vi "ExecuteSequence.vi"(8 "error in (no error)":errorcluster, 11 "Sequence in":refnum<class "Sequence.lvclass">) -> (0 "error out":errorcluster, 1 "Command":string, 2 "SweepProperties":T1, 3 "Sequence out":refnum<class "Sequence.lvclass">, 4 "Sequence is done":bool, 6 "Next Position":T4)   [LabVIEW 2018, in "Sequence.lvclass"]
uses:
  Sequence.lvclass
  SequenceSubvis/PatchNewTestStep.ctl
  SequenceSubvis/RF Direction.ctl
  SequenceSubvis/PolarizationSelect.ctl
  APARMainSubvis/VXM Public API/singleAxisMoveDef.ctl
  APARMainSubvis/VXM Public API/mmWaveAxis.ctl
  Datalog/DatalogSubvis/SearchableTag.ctl
  Support/MessageAPI/UIMessage.ctl
  Sequence.lvclass/Sequence.ctl
  SendMessage/SendMessage.lvclass
  Datalog/DataLog.lvclass
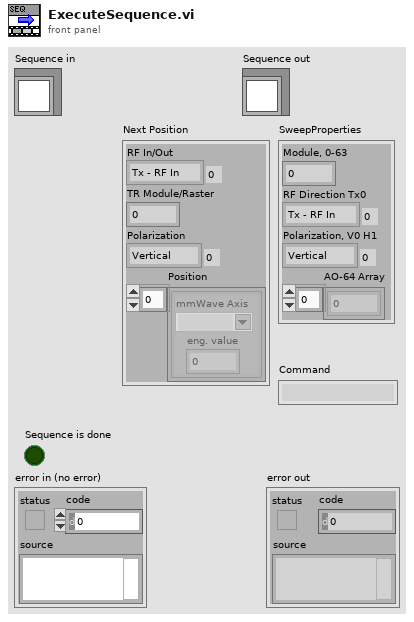
[diagram p1: front panel]
types:
  T1 = typedef "DataLog.lvclass/SearchableTag.ctl" = cluster{"Module, 0-63":i32, "RF Direction Tx0":T2, "Polarization, V0 H1":T3, "AO-64 Array":dbl[]}
  T2 = typedef "RF Direction.ctl" = enum16{"Tx - RF In", "Rx - RF Out"}
  T3 = typedef "PolarizationSelect.ctl" = enum16{"Vertical", "Horizontal"}
  T4 = typedef "PatchNewTestStep.ctl" = cluster{"RF In/Out":T2, "TR Module/Raster":i32, "Polarization":T3, "Position":T5[]}
  T5 = typedef "singleAxisMoveDef.ctl" = cluster{"mmWave Axis":T6, "eng. value":dbl}
  T6 = typedef "mmWaveAxis.ctl" = string
  T7 = typedef "UIMessage.ctl" = cluster{"EventCode":i32, "Numeric":dbl, "String":string, "Variant":variant}
  T8 = typedef "mWaveTestStep.ctl" = cluster{"StepType":T9, "RF In/Out":T2, "Module/Raster":i32, "Polarization":T3, "AO-64 Array":dbl[], "Position":T5[]}
  T9 = typedef "TestStepTypes.ctl" = enum16{"MotionFF-M2", "Motion", "SweepTest", "RasterTest", "Finish", "64ModuleCfg"}
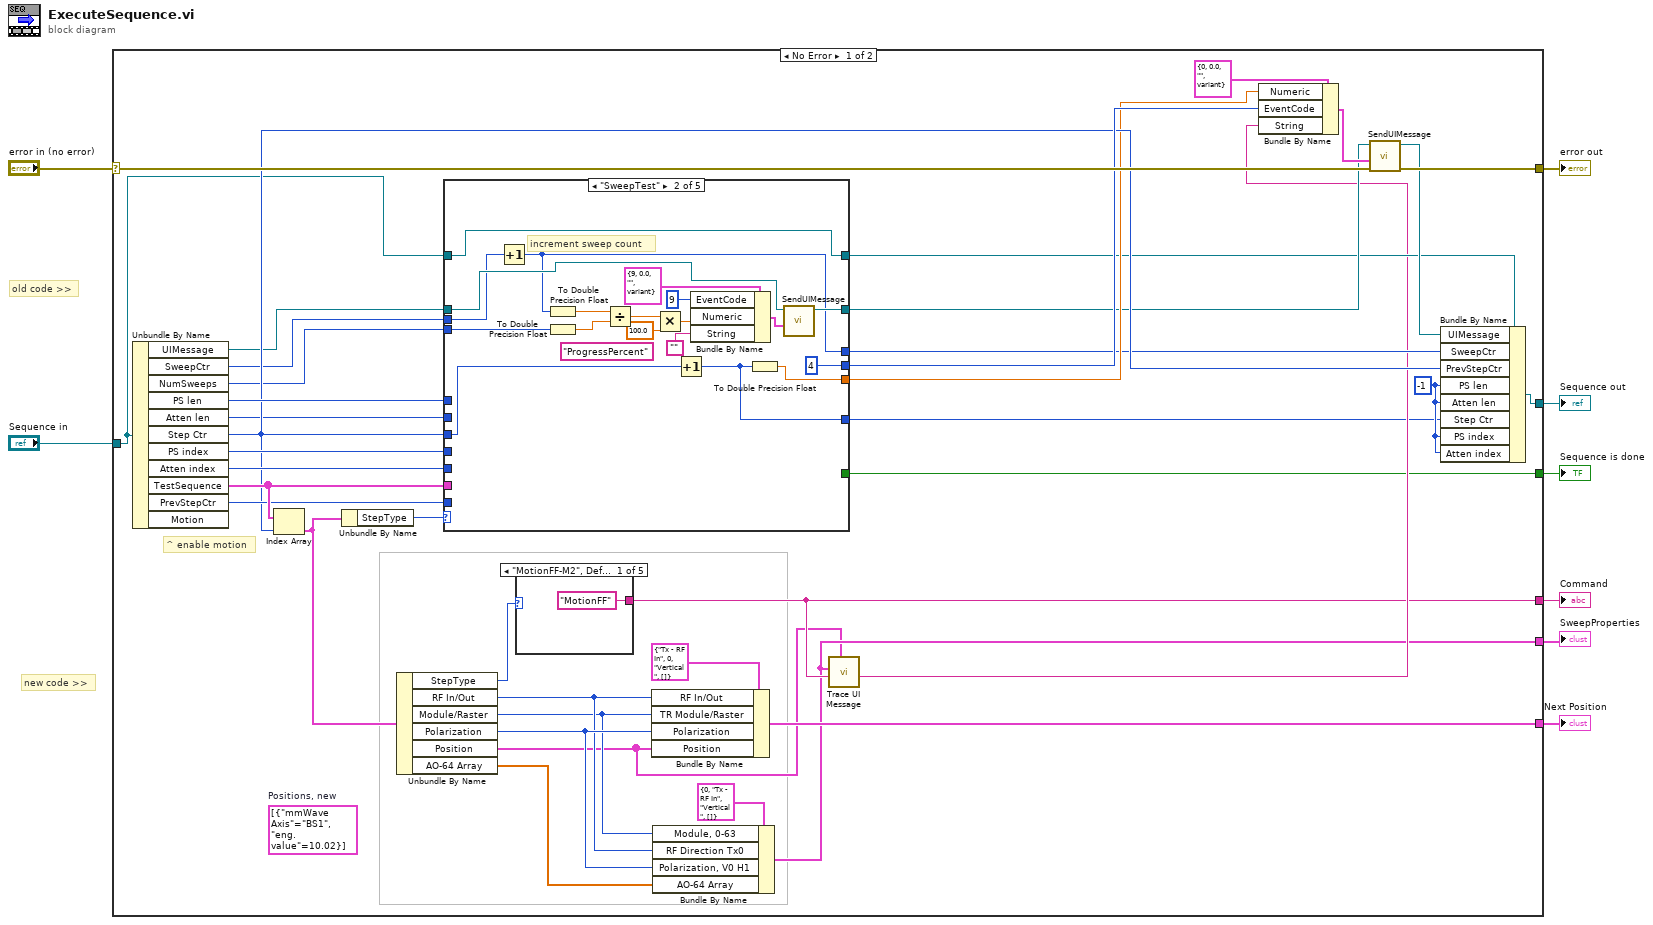
[diagram p0: block diagram]
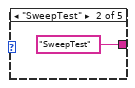
[diagram p2: hidden frame]
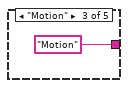
[diagram p3: hidden frame]
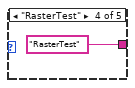
[diagram p4: hidden frame]
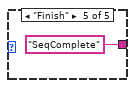
[diagram p5: hidden frame]
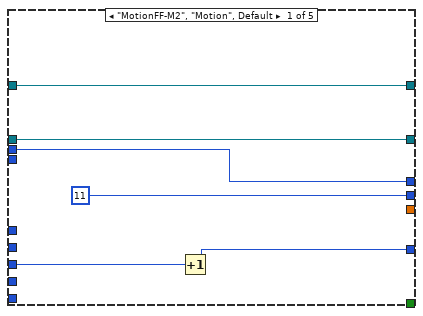
[diagram p6: hidden frame]
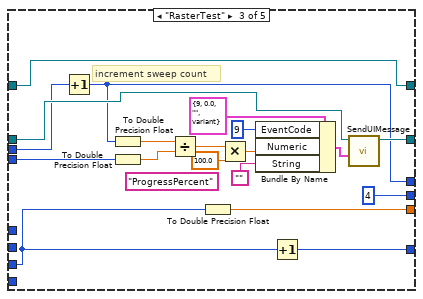
[diagram p7: hidden frame]
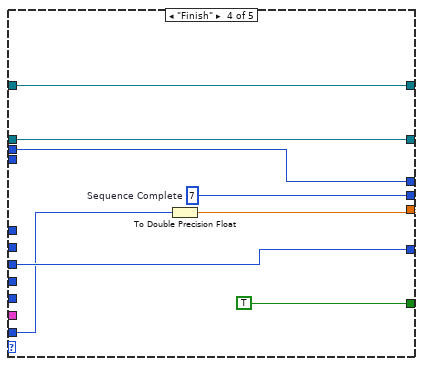
[diagram p8: hidden frame]
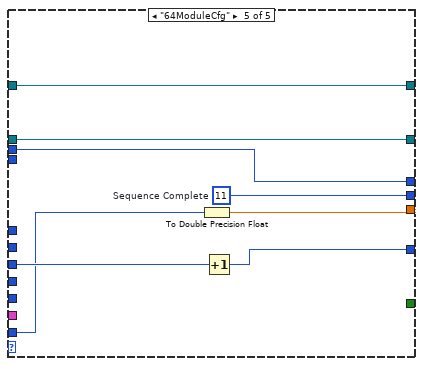
[diagram p9: hidden frame]
diagram:
  # "new code >>"
  # "old code >>"
  n1 = case shown="No Error" "error in (no error)" {
    selector: "error in (no error)" -> [w39 w114]
    tunnel: [w40 w114] -> w7
    tunnel: [w47 w113] -> w5
    tunnel: "Sequence in" -> [w26 w113]
    tunnel: [w12 _] -> w4
    tunnel: [w22 _] -> w3
    tunnel: [w13 _] -> w2
    tunnel: [w11 _] -> w1
    frame No Error {
      (unwired) T5[] [{"mmWave Axis"="BS1", "eng. value"=10.02}]  # Positions, new
      w23 = -1 ("Execution.PS len")
      # "^ enable motion"
      n2 = Unbundle By Name(w26) -> ("UIMessage"=w29:refnum<class "SendMessage.lvclass">, "SweepCtr"=w32:i32, "NumSweeps"=w31:i32, "PS len"=w46:i32, "Atten len"=w34:i32, "Step Ctr"=w35:i32, "PS index"=w45:i32, "Atten index"=w43:i32, "TestSequence"=w44:T8[], "PrevStepCtr"=w36:i32)  [unwired: 1 out]
      n3 = Index Array(array=w44, index=w35) -> (element=w14:T8)
      n4 = Unbundle By Name(w14) -> ("StepType"=w42:T9)
      n5 = Unbundle By Name(w14) -> ("StepType"=w20:T9, "RF In/Out"=w18:T2, "Module/Raster"=w17:i32, "Polarization"=w19:T3, "Position"=w9:T5[], "AO-64 Array"=w10:dbl[])
      n6 = case shown="\"SweepTest\"" w42 {
        tunnel: w45 -> [_ _ _ _ _]
        tunnel: w43 -> [_ _ _ _ _]
        tunnel: w46 -> [_ _ _ _ _]
        tunnel: w35 -> [w54 w76 w94 w102 w110]
        tunnel: [w53 w59 w96 w102 w105] -> w21
        tunnel: w44 -> [_ _ _ _ _]
        tunnel: [11 ("EventCode") 4 ("EventCode") 4 ("EventCode") w104 w112] -> w37
        tunnel: w36 -> [_ _ _ w101 w109]
        tunnel: w34 -> [_ _ _ _ _]
        tunnel: [_ w75 w93 w103 w111] -> w33
        tunnel: w32 -> [w57 w64 w82 w100 w108]
        tunnel: w31 -> [_ w70 w88 _ _]
        tunnel: [w57 w63 w81 w100 w108] -> w30
        tunnel: w29 -> [w56 w65 w83 w99 w107]
        tunnel: [w56 w69 w87 w99 w107] -> w28
        tunnel: w26 -> [w55 w60 w78 w98 w106]
        tunnel: [w55 w60 w78 w98 w106] -> w25
        tunnel: [_ _ _ TRUE _] -> w22
        frame "MotionFF-M2", "Motion", Default {
          n7 = Increment(x=w54) -> (x+1=w53:i32)
        }
        frame "SweepTest" {
          (unwired) "ProgressPercent" ("String")
          # "increment sweep count"
          n8 = Increment(x=w64) -> (x+1=w63:i32)
          n9 = To Double Precision Float(number=w63) -> (double precision float=w73:dbl)
          n10 = To Double Precision Float(number=w70) -> (double precision float=w72:dbl)
          n11 = Divide(x=w73, y=w72) -> (x/y=w68:dbl)
          n12 = Multiply(x=w68, y=100.0) -> (x*y=w66:dbl)
          n13 = Increment(x=w76) -> (x+1=w59:i32)
          n14 = Bundle By Name(cluster=T7 {"EventCode"=9, "Numeric"=0.0, "String"="", "Variant"=variant} ("UIMsg"), "EventCode"=9, "Numeric"=w66, "String"="") -> (w71:T7)
          n15 = To Double Precision Float(number=w59) -> (double precision float=w75:dbl)
          n16 = call-dynamic "SendUIMessage.vi"("UIMsg"=w71, "SendMessage in"=w65) -> ("SendMessage out"=w69:refnum<class "SendMessage.lvclass">)  [unwired: 8 in, 1 out]
        }
        frame "RasterTest" {
          (unwired) "ProgressPercent" ("String")
          # "increment sweep count"
          n17 = Increment(x=w82) -> (x+1=w81:i32)
          n18 = To Double Precision Float(number=w81) -> (double precision float=w91:dbl)
          n19 = To Double Precision Float(number=w88) -> (double precision float=w90:dbl)
          n20 = Divide(x=w91, y=w90) -> (x/y=w86:dbl)
          n21 = To Double Precision Float(number=w94) -> (double precision float=w93:dbl)
          n22 = Multiply(x=w86, y=100.0) -> (x*y=w84:dbl)
          n23 = Bundle By Name(cluster=T7 {"EventCode"=9, "Numeric"=0.0, "String"="", "Variant"=variant} ("UIMsg"), "EventCode"=9, "Numeric"=w84, "String"="") -> (w89:T7)
          n24 = Increment(x=w94) -> (x+1=w96:i32)
          n25 = call-dynamic "SendUIMessage.vi"("UIMsg"=w89, "SendMessage in"=w83) -> ("SendMessage out"=w87:refnum<class "SendMessage.lvclass">)  [unwired: 8 in, 1 out]
        }
        frame "Finish" {
          w104 = 7  # Sequence Complete
          n26 = To Double Precision Float(number=w101) -> (double precision float=w103:dbl)
        }
        frame "64ModuleCfg" {
          w112 = 11  # Sequence Complete
          n27 = To Double Precision Float(number=w109) -> (double precision float=w111:dbl)
          n28 = Increment(x=w110) -> (x+1=w105:i32)
        }
      }
      n29 = case shown="\"MotionFF-M2\", Default" w20 {
        tunnel: ["MotionFF" ("Command") "SweepTest" ("Command") "Motion" ("Command") "RasterTest" ("Command") "SeqComplete" ("Command")] -> w13
        frame "MotionFF-M2", Default {
        }
        frame "SweepTest" {
        }
        frame "Motion" {
        }
        frame "RasterTest" {
        }
        frame "Finish" {
        }
      }
      n30 = Bundle By Name(cluster=T4 {"RF In/Out"=enum."Tx - RF In", "TR Module/Raster"=0, "Polarization"=enum."Vertical", "Position"=[]} ("NewSetup"), "RF In/Out"=w18, "TR Module/Raster"=w17, "Polarization"=w19, "Position"=w9) -> (w12:T4)
      n31 = Bundle By Name(cluster=T1 {"Module, 0-63"=0, "RF Direction Tx0"=enum."Tx - RF In", "Polarization, V0 H1"=enum."Vertical", "AO-64 Array"=[]} ("SweepProperties"), "Module, 0-63"=w17, "RF Direction Tx0"=w18, "Polarization, V0 H1"=w19, "AO-64 Array"=w10) -> (w11:T1)
      n32 = call "Trace UI Message.vi"("Position"=w9, "Command"=w13, "SweepProperties"=w11) -> ("UI Msg String"=w24:string)  [unwired: 8 in]
      n33 = Bundle By Name(cluster=T7 {"EventCode"=0, "Numeric"=0.0, "String"="", "Variant"=variant} ("UIMsg"), "Numeric"=w33, "EventCode"=w37, "String"=w24) -> (w38:T7)
      n34 = call-dynamic "SendUIMessage.vi"("error in (no error)"=w39, "UIMsg"=w38, "SendMessage in"=w28) -> ("error out"=w40:errorcluster, "SendMessage out"=w27:refnum<class "SendMessage.lvclass">)  [unwired: 7 in]
      n35 = Bundle By Name(cluster=w25, "UIMessage"=w27, "SweepCtr"=w30, "PrevStepCtr"=w35, "PS len"=w23, "Atten len"=w23, "Step Ctr"=w21, "PS index"=w23, "Atten index"=w23) -> (w47:refnum<class "Sequence.lvclass">)
    }
    frame Error {
    }
  }
  "error out" <- w7
  "Sequence out" <- w5
  "Next Position" <- w4
  "Sequence is done" <- w3
  "Command" <- w2
  "SweepProperties" <- w1
